vi "GPS~Logger.vi"(0 "VISA resource name":refnum<visa-resource-name>, 1 "stop":bool, 2 "baud rate (115200)":u32=115200, 3 "file path (use dialog)":path, 4 "Camera Log":bool=TRUE) -> (5 "Lattitude":dbl format="%#_15g", 6 "Longitude":dbl format="%#_15g")   [LabVIEW 2010]
uses:
  <vilib>/robotics/Controls/Attitude Indicator/Attitude Indicator.xctl
  <vilib>/robotics/Controls/Compass Indicator/Compass Indicator.xctl
  <vilib>/Instr/_visa.llb/VISA Set IO Buffer Mask.ctl
  <vilib>/Instr/_visa.llb/VISA Configure Serial Port (Instr).vi
panel:
  out "Present Text":string
  out "String":string
  out "Bearing":dbl
  out "Speed":dbl(knob) scale=0.0..40.0
  out "LiPo":i32(slide) scale=9.0..12.6
  out "GPS Time":string
  out "Servo Roll":string
  out "Battery Voltage":dbl
  out "Distance to Waypoint":string
  out "Waypoint Number":string
  out "Flight Mode":string
  out "Compass Indicator":dbl(xcontrol)
  out "Attitude Indicator":cluster{"Roll":dbl, "Pitch":dbl}(xcontrol)
  out "Message Text":string
  in  "Tab Control":enum32{"Connectivity", "Attitude", "GPS"}(tab)
  out "error out":errorcluster {"code" format="%f"}
  out "Roll":string
  out "Pitch":string
  out "Throttle":string
  out "Airspeed":string
  out "Roll Pitch":cluster{dbl, dbl}
  out "YawNum":dbl
  out "ALT":string
  out "ALH":string
  out "BER":string
  out "CRT":string
  out "SPD":string
  out "CRS":string
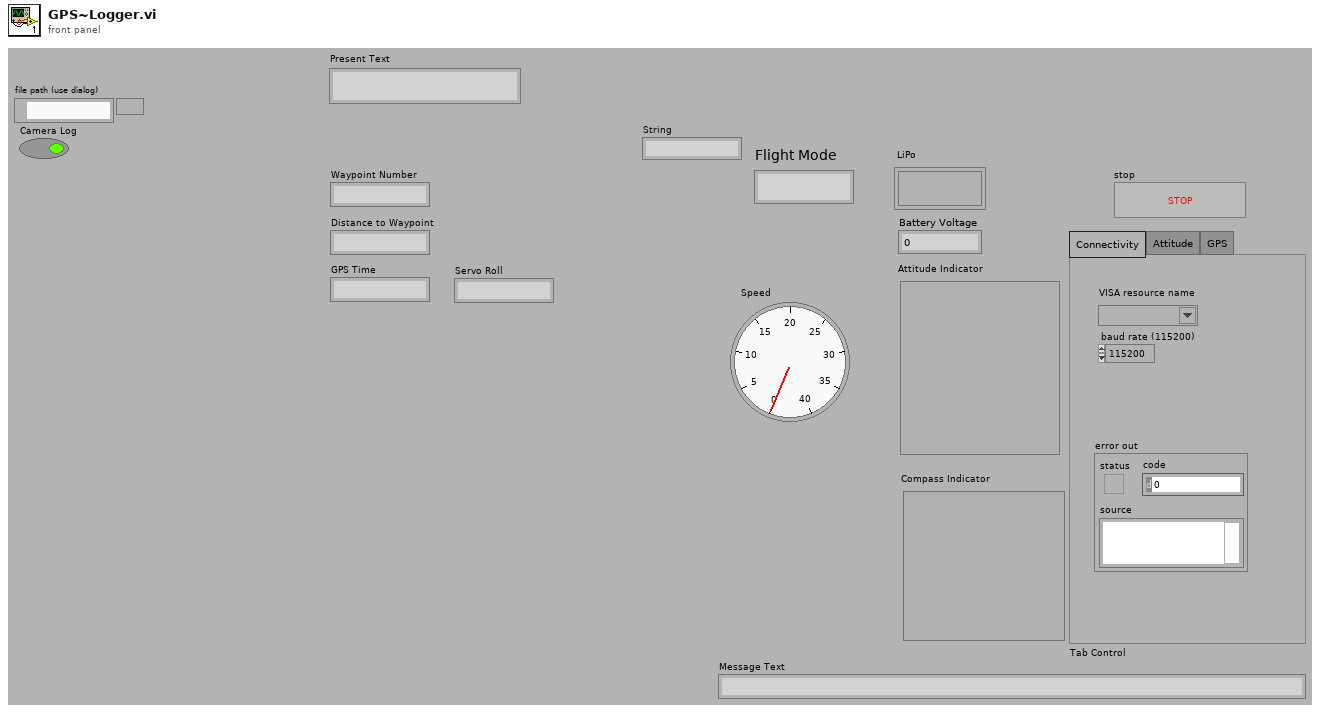
[diagram p1: front panel]
types:
  T1 = typedef "VISA Set IO Buffer Mask.ctl" = u16
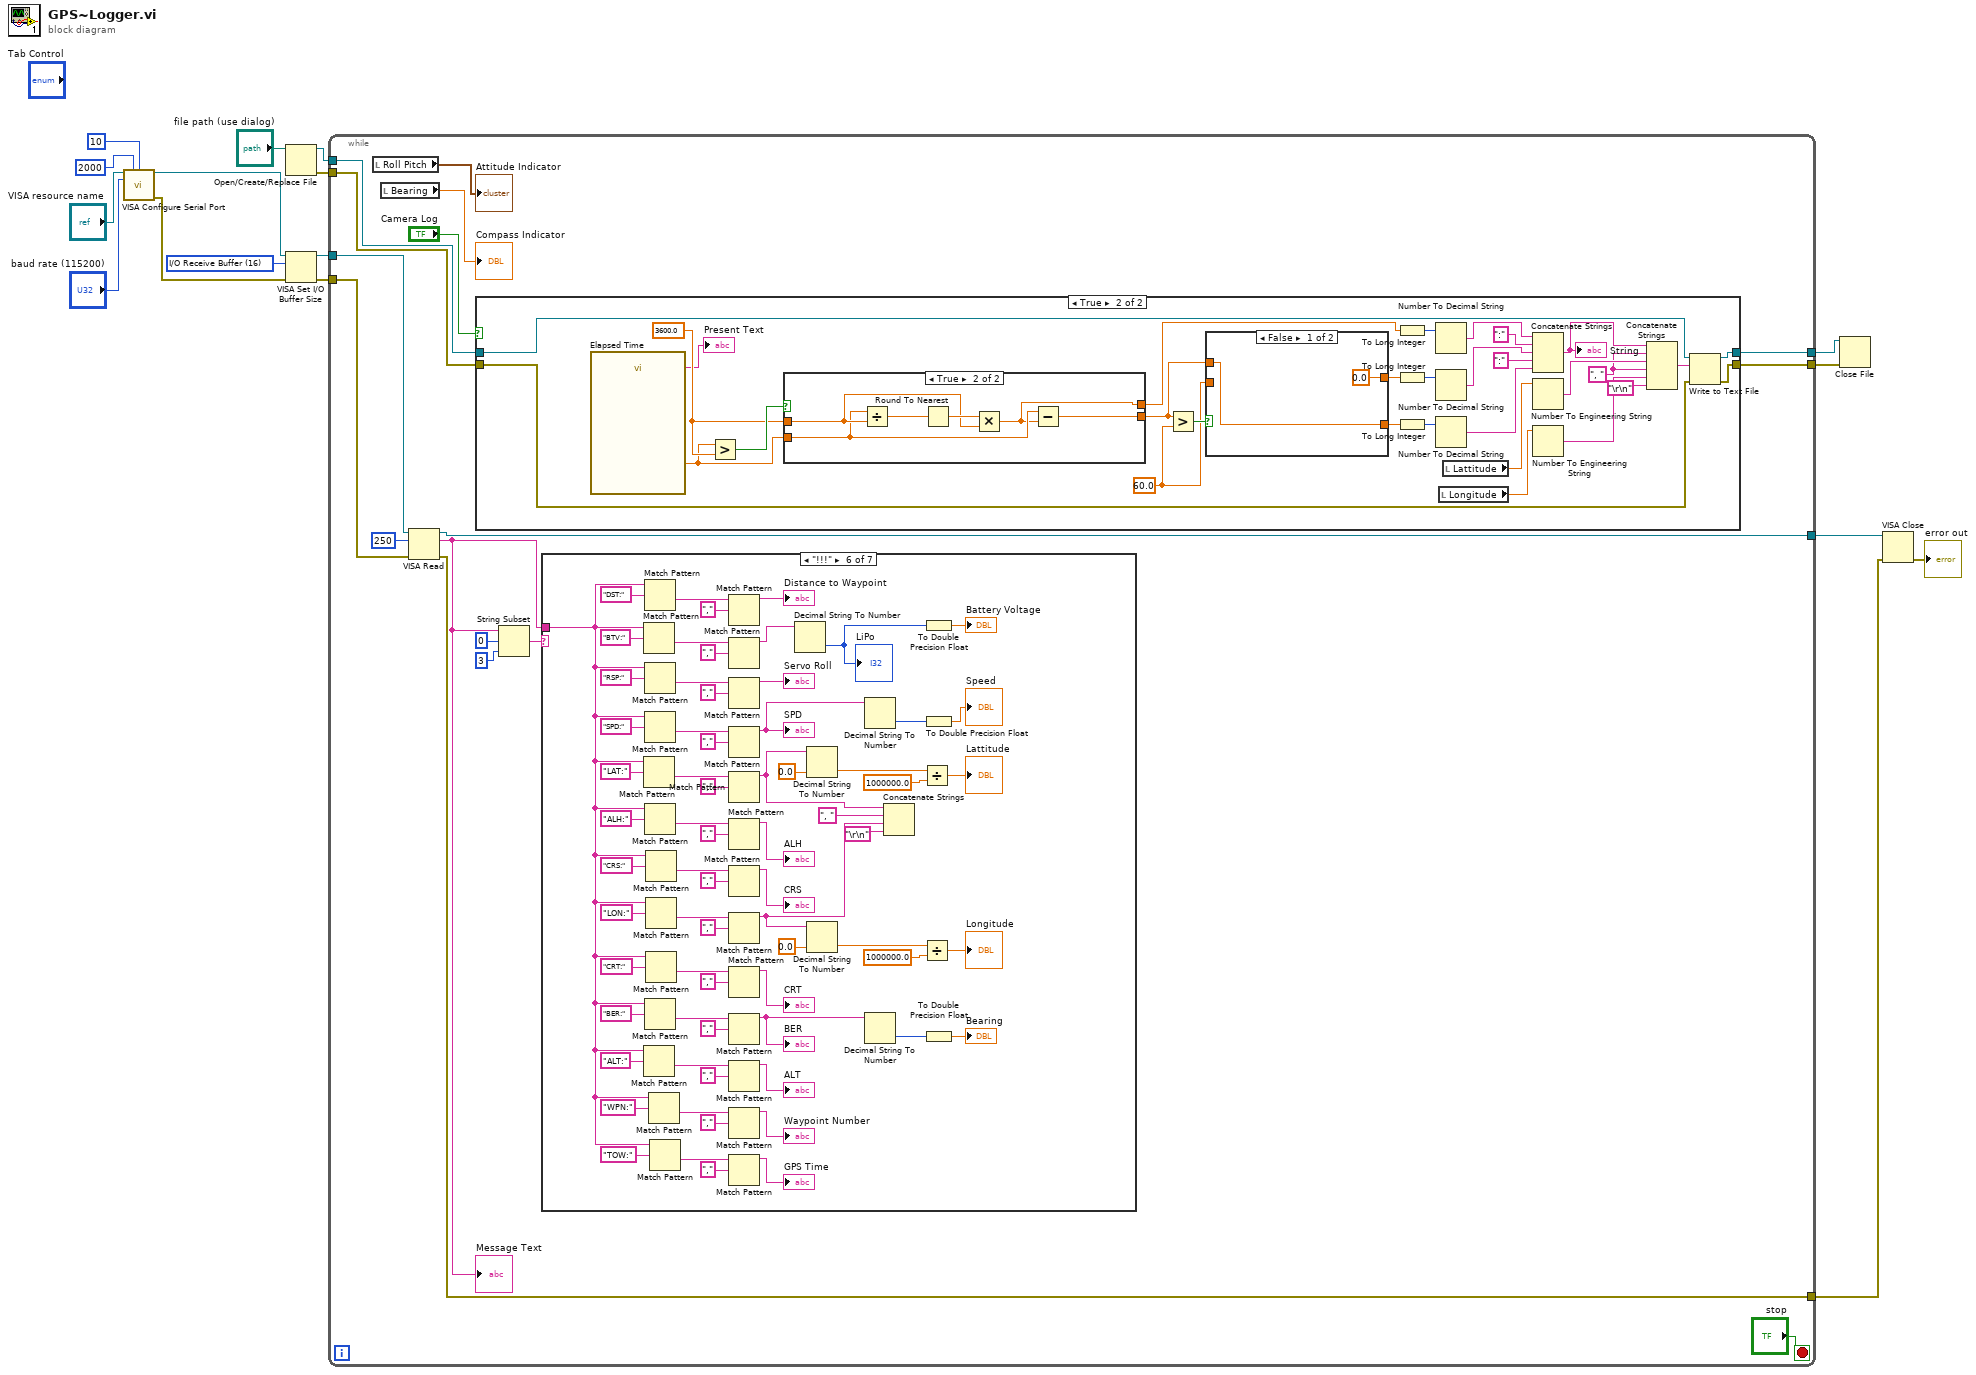
[diagram p0: block diagram]
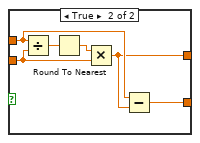
[diagram p3: hidden frame]
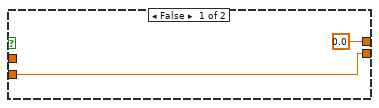
[diagram p4: hidden frame]
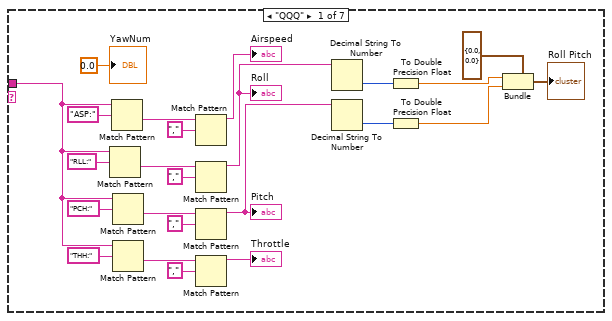
[diagram p5: hidden frame]
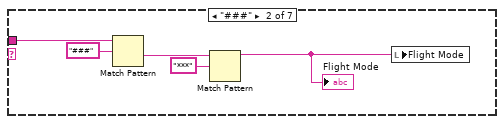
[diagram p6: hidden frame]
diagram:
  w12 = T1 16 items=["I/O Receive Buffer"=16, "I/O Transmit Buffer"=32, "I/O Receive and Transmit Buffer"=48] ("Mask")
  n1 = call-poly "VISA Configure Serial Port"("VISA resource name"="VISA resource name", "timeout (10sec)"=u32 2000, "termination char\n(0xA = '\\n' = LF)"=u8 10 ("termination char\n(0xA = '\\n' = LF)"), "baud rate (9600)"="baud rate (115200)") -> ("VISA resource name out"=w13:refnum<visa-resource-name>, "error out"=w7:errorcluster)  [unwired: 10 in]
  n2 = Open/Create/Replace File(file path (use dialog)="file path (use dialog)") -> (refnum out=w5:refnum<file>, error out=w1:errorcluster)  [unwired: 5 in, 1 out]
  n3 = VISA Set I/O Buffer Size(VISA resource name=w13, mask (16)=w12, error in (no error)=w7) -> (VISA resource name out=w11:refnum<visa-resource-name>, error out=w8:errorcluster)  [unwired: 1 in]
  n4 = while {
    tunnel: w11 -> [w34]
    tunnel: [w32] -> w10
    tunnel: [w31] -> w9
    tunnel: w8 -> [w30]
    tunnel: w5 -> [w22]
    tunnel: [w21] -> w3
    tunnel: [w20] -> w2
    tunnel: w1 -> [w19]
    stop <- "stop" stop-if-true
    n5 = local read "Roll Pitch"() -> (→"Attitude Indicator":cluster{dbl, dbl})
    n6 = local read "Bearing"() -> (→"Compass Indicator":dbl)
    n7 = VISA Read(VISA resource name=w34, byte count=u32 250, error in (no error)=w30) -> (VISA resource name out=w32:refnum<visa-resource-name>, read buffer=w24:string, error out=w31:errorcluster)  [unwired: 1 out]
    "Message Text" <- w24
    n8 = case shown="True" "Camera Log" {
      tunnel: w22 -> [w36 w66]
      tunnel: [w36 w65] -> w21
      tunnel: [w35 w63] -> w20
      tunnel: w19 -> [w35 w62]
      frame False {
      }
      frame True {
        w43 = 60.0 ("y")
        w45 = 3600.0 ("y")
        w57 = ", " ("string")
        n9 = call "Elapsed Time"() -> ("Present Text"=→"Present Text":string, "Elapsed Time (s)"=w40:dbl)  [unwired: 12 in, 6 out]
        n10 = Greater?(x=w40, y=w45) -> (0:w46:bool)
        n11 = case shown="True" w46 {
          tunnel: w40 -> [w76 w79]
          tunnel: w45 -> [_ w81]
          tunnel: [w76 w78] -> w42
          tunnel: [0.0 w77] -> w39
          frame False {
          }
          frame True {
            n12 = Divide(x=w79, y=w81) -> (x/y=w80:dbl)
            n13 = Round To Nearest(number=w80) -> (nearest integer value=w82:dbl)
            n14 = Multiply(x=w82, y=w81) -> (x*y=w77:dbl)
            n15 = Subtract(x=w79, y=w77) -> (x-y=w78:dbl)
          }
        }
        n16 = Greater?(x=w42, y=w43) -> (0:w44:bool)
        n17 = case shown="False" w44 {
          tunnel: w42 -> [w68 w71]
          tunnel: w43 -> [_ w73]
          tunnel: [w68 w70] -> w38
          tunnel: [0.0 w69] -> w37
          frame False {
          }
          frame True {
            n18 = Divide(x=w71, y=w73) -> (x/y=w72:dbl)
            n19 = Round To Nearest(number=w72) -> (nearest integer value=w74:dbl)
            n20 = Multiply(x=w74, y=w73) -> (x*y=w69:dbl)
            n21 = Subtract(x=w71, y=w69) -> (x-y=w70:dbl)
          }
        }
        n22 = To Long Integer(number=w39) -> (32bit integer=w56:i32)
        n23 = To Long Integer(number=w37) -> (32bit integer=w55:i32)
        n24 = To Long Integer(number=w38) -> (32bit integer=w54:i32)
        n25 = Number To Decimal String(number=w56) -> (decimal integer string=w53:string)  [unwired: 1 in]
        n26 = Number To Decimal String(number=w55) -> (decimal integer string=w52:string)  [unwired: 1 in]
        n27 = Number To Decimal String(number=w54) -> (decimal integer string=w51:string)  [unwired: 1 in]
        n28 = local read "Longitude"() -> (w61:dbl)
        n29 = local read "Lattitude"() -> (w58:dbl)
        n30 = Concatenate Strings(w53, ":" ("string"), w52, ":" ("string"), w51) -> (w47:string)
        "String" <- w47
        n31 = Number To Engineering String(4:w58) -> (0:w59:string)  [unwired: 3 in]
        n32 = Number To Engineering String(4:w61) -> (0:w60:string)  [unwired: 3 in]
        n33 = Concatenate Strings(w47, w57, w59, w57, w60, "\r\n") -> (w64:string)
        n34 = Write to Text File(file (use dialog)=w66, text=w64, error in=w62) -> (refnum out=w65:refnum<file>, error out=w63:errorcluster)  [unwired: 1 in, 1 out]
      }
    }
    n35 = String Subset(string=w24, offset (0)=0, length (rest)=3 ("length (rest)")) -> (substring=w23:string)
    n36 = case shown="\"!!!\"" w23 {
      tunnel: w24 -> [w84 w111 _ _ _ w132 _]
      frame "QQQ" {
        n37 = Match Pattern(string=w84, regular expression="RLL:") -> (after substring=w105:string)  [unwired: 4 out]
        n38 = Match Pattern(string=w84, regular expression="ASP:") -> (after substring=w96:string)  [unwired: 4 out]
        n39 = Match Pattern(string=w84, regular expression="PCH:") -> (after substring=w102:string)  [unwired: 4 out]
        n40 = Match Pattern(string=w84, regular expression="THH:") -> (after substring=w99:string)  [unwired: 4 out]
        n41 = Match Pattern(string=w96, regular expression=",") -> (before substring=→"Airspeed":string)  [unwired: 4 out]
        n42 = Match Pattern(string=w105, regular expression=",") -> (before substring=w87:string)  [unwired: 4 out]
        "Roll" <- w87
        n43 = Match Pattern(string=w102, regular expression=",") -> (before substring=w86:string)  [unwired: 4 out]
        "Pitch" <- w86
        n44 = Match Pattern(string=w99, regular expression=",") -> (before substring=→"Throttle":string)  [unwired: 4 out]
        n45 = Decimal String To Number(string=w87) -> (number=w93:i32)  [unwired: 2 in, 1 out]
        n46 = Decimal String To Number(string=w86) -> (number=w92:i32)  [unwired: 2 in, 1 out]
        n47 = To Double Precision Float(number=w93) -> (double precision float=w90:dbl)
        n48 = To Double Precision Float(number=w92) -> (double precision float=w91:dbl)
        n49 = Bundle(cluster=cluster{dbl, dbl} {0.0, 0.0} ("Cluster"), w90, w91) -> (→"Roll Pitch":cluster{dbl, dbl})
        "YawNum" <- 0.0 ("YawNum")
      }
      frame "###" {
        n50 = Match Pattern(string=w111, regular expression="###") -> (after substring=w109:string)  [unwired: 1 in, 3 out]
        n51 = Match Pattern(string=w109, regular expression="***") -> (before substring=w107:string)  [unwired: 1 in, 3 out]
        "Flight Mode" <- w107
        n52 = local write "Flight Mode"(w107) -> ()
      }
      frame "%%%" {
      }
      frame "XXX" {
      }
      frame "PPP" {
      }
      frame "!!!" {
        n53 = Match Pattern(string=w132, regular expression="BTV:") -> (after substring=w142:string)  [unwired: 4 out]
        n54 = Match Pattern(string=w132, regular expression="LAT:") -> (after substring=w179:string)  [unwired: 4 out]
        n55 = Match Pattern(string=w132, regular expression="ALT:") -> (after substring=w173:string)  [unwired: 4 out]
        n56 = Match Pattern(string=w132, regular expression="DST:") -> (after substring=w146:string)  [unwired: 4 out]
        n57 = Match Pattern(string=w132, regular expression="RSP:") -> (after substring=w139:string)  [unwired: 4 out]
        n58 = Match Pattern(string=w132, regular expression="SPD:") -> (after substring=w169:string)  [unwired: 4 out]
        n59 = Match Pattern(string=w132, regular expression="ALH:") -> (after substring=w156:string)  [unwired: 4 out]
        n60 = Match Pattern(string=w132, regular expression="BER:") -> (after substring=w159:string)  [unwired: 4 out]
        n61 = Match Pattern(string=w132, regular expression="CRS:") -> (after substring=w162:string)  [unwired: 4 out]
        n62 = Match Pattern(string=w132, regular expression="LON:") -> (after substring=w176:string)  [unwired: 4 out]
        n63 = Match Pattern(string=w132, regular expression="CRT:") -> (after substring=w166:string)  [unwired: 4 out]
        n64 = Match Pattern(string=w132, regular expression="WPN:") -> (after substring=w150:string)  [unwired: 4 out]
        n65 = Match Pattern(string=w132, regular expression="TOW:") -> (after substring=w135:string)  [unwired: 4 out]
        n66 = Match Pattern(string=w146, regular expression=",") -> (before substring=→"Distance to Waypoint":string)  [unwired: 4 out]
        n67 = Match Pattern(string=w142, regular expression=",") -> (before substring=w131:string)  [unwired: 4 out]
        n68 = Match Pattern(string=w139, regular expression=",") -> (before substring=→"Servo Roll":string)  [unwired: 4 out]
        n69 = Match Pattern(string=w169, regular expression=",") -> (before substring=w126:string)  [unwired: 4 out]
        "SPD" <- w126
        n70 = Match Pattern(string=w179, regular expression=",") -> (before substring=w121:string)  [unwired: 4 out]
        n71 = Match Pattern(string=w156, regular expression=",") -> (before substring=→"ALH":string)  [unwired: 4 out]
        n72 = Match Pattern(string=w162, regular expression=",") -> (before substring=→"CRS":string)  [unwired: 4 out]
        n73 = Match Pattern(string=w176, regular expression=",") -> (before substring=w117:string)  [unwired: 4 out]
        n74 = Match Pattern(string=w166, regular expression=",") -> (before substring=→"CRT":string)  [unwired: 4 out]
        n75 = Match Pattern(string=w159, regular expression=",") -> (before substring=w122:string)  [unwired: 4 out]
        "BER" <- w122
        n76 = Match Pattern(string=w173, regular expression=",") -> (before substring=→"ALT":string)  [unwired: 4 out]
        n77 = Match Pattern(string=w150, regular expression=",") -> (before substring=→"Waypoint Number":string)  [unwired: 4 out]
        n78 = Match Pattern(string=w135, regular expression=",") -> (before substring=→"GPS Time":string)  [unwired: 4 out]
        n79 = Decimal String To Number(string=w131) -> (number=w129:i32)  [unwired: 2 in, 1 out]
        "LiPo" <- w129
        n80 = Decimal String To Number(string=w121, default (0L)=0.0 ("default (0 I32)")) -> (number=w114:dbl)  [unwired: 1 in, 1 out]
        n81 = Decimal String To Number(string=w117, default (0L)=0.0 ("default (0 I32)")) -> (number=w112:dbl)  [unwired: 1 in, 1 out]
        n82 = Decimal String To Number(string=w126) -> (number=w127:i32)  [unwired: 2 in, 1 out]
        n83 = Decimal String To Number(string=w122) -> (number=w125:i32)  [unwired: 2 in, 1 out]
        n84 = Concatenate Strings(w121, ", " ("string"), w117, "\r\n") -> ()  [unwired: 1 out]
        n85 = Divide(x=w114, y=1000000.0) -> (x/y=→"Lattitude":dbl)
        n86 = Divide(x=w112, y=1000000.0) -> (x/y=→"Longitude":dbl)
        n87 = To Double Precision Float(number=w129) -> (double precision float=→"Battery Voltage":dbl)
        n88 = To Double Precision Float(number=w127) -> (double precision float=→"Speed":dbl)
        n89 = To Double Precision Float(number=w125) -> (double precision float=→"Bearing":dbl)
      }
      frame Default {
      }
    }
  }
  n90 = Close File(refnum=w3, error in=w2) -> ()  [unwired: 2 out]
  n91 = VISA Close(VISA resource name=w10, error in (no error)=w9) -> (error out=→"error out":errorcluster)
